vi "NR Example.vi"() -> ()   [LabVIEW 2016]
uses:
  Source/SA/RFmxNR/Typedefs/NR Common Configuration.ctl
  Source/SA/RFmxNR/Typedefs/NR Signal Configuration.ctl
  Source/SA/RFmxNR/Typedefs/NR ModAcc Configuration.ctl
  Source/SA/RFmxNR/Typedefs/NR ACP Configuration.ctl
  Source/SA/RFmxNR/Typedefs/NR ModAcc Results.ctl
  Source/SA/RFmxNR/Typedefs/NR ModAcc Component Carrier Results.ctl
  Source/SA/RFmxNR/Typedefs/NR ACP Results.ctl
  Source/SA/RFmxNR/Typedefs/NR ACP Offset Results.ctl
  Source/SA/RFmxNR/Typedefs/NR ACP Component Carrier Results.ctl
  Source/SA/RFmxNR/Typedefs/NR CHP Configuration.ctl
  Source/SA/RFmxNR/Typedefs/NR CHP Results.ctl
  Source/SA/RFmxNR/Typedefs/NR CHP Component Carrier Results.ctl
  Source/SA/RFmxNR/RFmxNR.lvlib
panel:
  out "CHP Results":T1
  out "error out":errorcluster
  out "ACP Results":T3
  out "ModAcc Results":T6
  in  "Tab Control":T8(tab)=enum."CHP"
  in  "Common Configuration":T9={"Center Frequency (Hz)"=3500000000.0, "Reference Level (dBm)"=0.0, "External Attenuation (dB)"=0.0, "Frequency Reference Source"="PXI_Clk", "Enable Trigger?"=TRUE, "Digital Edge Source"="PXI_Trig0", "Digital Edge Type"=0, "Trigger Delay (s)"=0.0, "Auto Level Enabled?"=FALSE, "Auto Level Measurement Interval (s)"=0.01} {"Auto Level Measurement Interval (s)" format="%.3p"; "Trigger Delay (s)" format="%.3p"; "Digital Edge Type" items=["Rising Edge", "Falling Edge"]; "External Attenuation (dB)" format="%.2f"; "Reference Level (dBm)" format="%.2f"; "Center Frequency (Hz)" format="%.6p"}
  in  "Resource Name":refnum<k15>="VST2_01"
  in  "Signal Configuration":T10={"Link Direction"=1, "Frequency Range"=0, "Band"=78, "Auto Resource Block Detection Enabled"=1, "Component Carrier Configurations"=[{"Bandwidth (Hz)"=100000000.0, "Cell ID"=0, "PUSCH Modulation Type"=1, "Subcarrier Spacing (Hz)"=30000.0, "PUSCH Resource Block Offset"=0, "PUSCH Number of Resource Blocks"=-1, "PUSCH Transform Precoding Enabled"=0, "PUSCH Slot Allocation"="0-Last", "PUSCH Symbol Allocation"="0-Last", "PUSCH DMRS Configuration Type"=0, "PUSCH Mapping Type"=0, "PUSCH DMRS Type A Position"=2, "PUSCH DMRS Duration"=1, "PUSCH DMRS Additional Positions"=0}]} {"Component Carrier Configurations"."PUSCH DMRS Additional Positions" items=["0", "1", "2", "3"]; "Component Carrier Configurations"."PUSCH DMRS Duration" items=["Single-Symbol"=1, "Double-Symbol"=2]; "Component Carrier Configurations"."PUSCH DMRS Type A Position" items=["2"=2, "3"=3]; "Component Carrier Configurations"."PUSCH Mapping Type" items=["Type A", "Type B"]; "Component Carrier Configurations"."PUSCH DMRS Configuration Type" items=["Type 1", "Type 2"]; "Component Carrier Configurations"."PUSCH Transform Precoding Enabled" items=["False", "True"]; "Component Carrier Configurations"."Subcarrier Spacing (Hz)" items=["15kHz"=15000.0, "30kHz"=30000.0, "60kHz"=60000.0, "120kHz"=120000.0]; "Component Carrier Configurations"."PUSCH Modulation Type" items=["PI/2 BPSK", "QPSK", "16 QAM", "64 QAM", "256 QAM"]; "Component Carrier Configurations"."Bandwidth (Hz)" items=["5M"=5000000.0, "10M"=10000000.0, "15M"=15000000.0, "20M"=20000000.0, "25M"=25000000.0, "30M"=30000000.0, "40M"=40000000.0, "50M"=50000000.0, "60M"=60000000.0, "70M"=70000000.0, "80M"=80000000.0, "90M"=90000000.0, "100M"=100000000.0, "200M"=200000000.0, "400M"=400000000.0]; "Auto Resource Block Detection Enabled" items=["False", "True"]; "Frequency Range" items=["Range 1", "Range 2"]; "Link Direction" items=["Downlink", "Uplink"]}
  in  "ACP Configuration":T11={"Number of UTRA Offsets"=2, "Number of EUTRA Offsets"=0, "Number of NR Offsets"=1, "Number of ENDC Offsets"=0, "Measurement Method"=0, "Noise Compensation Enabled"=0, "Sweep Time Auto"=1, "Sweep Time Interval (s)"=0.001, "Averaging Enabled"=0, "Averaging Count"=10, "Averaging Type"=0} {"Measurement Method" items=["Normal", "Dynamic Range", "Sequential FFT"]; "Noise Compensation Enabled" items=["False", "True"]; "Sweep Time Auto" items=["False", "True"]; "Averaging Type" items=["RMS", "Log", "Scalar", "Max", "Min"]; "Averaging Enabled" items=["False", "True"]}
  in  "ModAcc Configuration":T12={"Measurement Length Unit"=1, "Measurement Offset"=0.0, "Measurement Length"=1.0, "EVM Unit"=0, "Averaging Enabled"=0, "Averaging Count"=10} {"Averaging Enabled" items=["False", "True"]; "EVM Unit" items=["Percentage", "dB"]; "Measurement Length Unit" items=["Slot"=1, "Subframe"=3, "Time"=6]}
  in  "CHP Configuration":T13={"Sweep Time Auto"=1, "Sweep Time Interval (s)"=0.001, "Averaging Enabled"=0, "Averaging Count"=10, "Averaging Type"=0} {"Sweep Time Auto" items=["False", "True"]; "Averaging Type" items=["RMS", "Log", "Scalar", "Max", "Min"]; "Averaging Enabled" items=["False", "True"]}
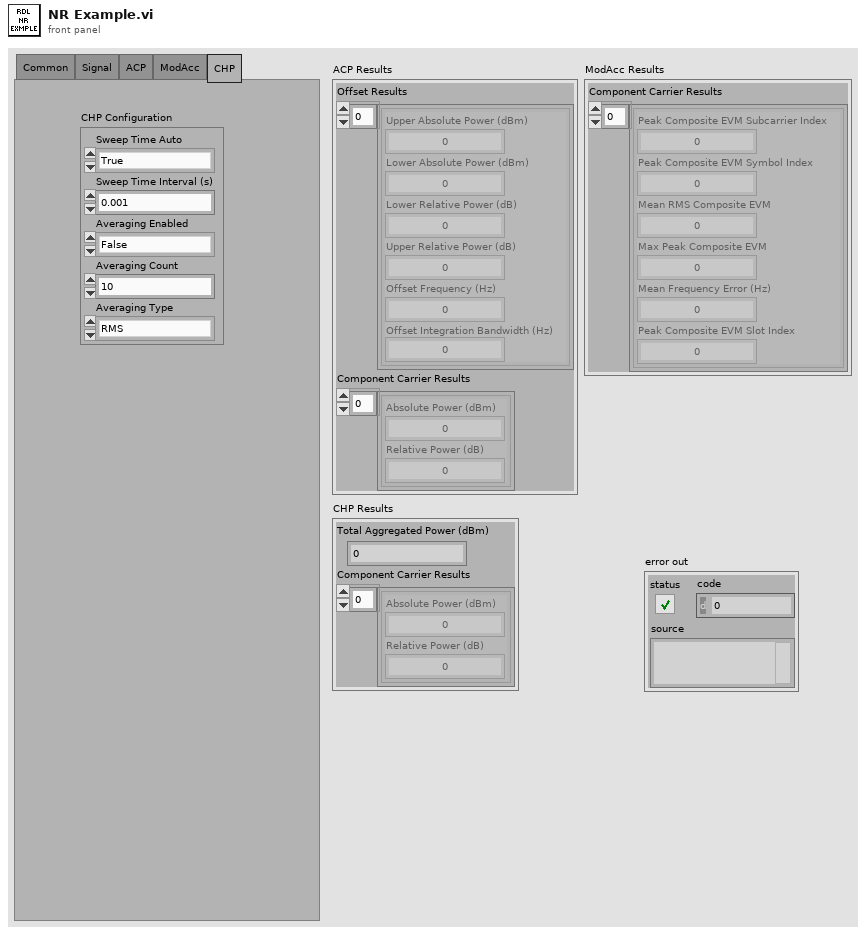
[diagram p1: front panel]
types:
  T1 = typedef "RFmxNR.lvlib/NR CHP Results.ctl" = cluster{"Total Aggregated Power (dBm)":dbl, "Component Carrier Results":T2[]}
  T2 = typedef "RFmxNR.lvlib/NR CHP Component Carrier Results.ctl" = cluster{"Absolute Power (dBm)":dbl, "Relative Power (dB)":dbl}
  T3 = typedef "RFmxNR.lvlib/NR ACP Results.ctl" = cluster{"Offset Results":T4[], "Component Carrier Results":T5[]}
  T4 = typedef "RFmxNR.lvlib/NR ACP Offset Results.ctl" = cluster{"Upper Absolute Power (dBm)":dbl, "Lower Absolute Power (dBm)":dbl, "Lower Relative Power (dB)":dbl, "Upper Relative Power (dB)":dbl, "Offset Frequency (Hz)":dbl, "Offset Integration Bandwidth (Hz)":dbl}
  T5 = typedef "RFmxNR.lvlib/NR ACP Component Carrier Results.ctl" = cluster{"Absolute Power (dBm)":dbl, "Relative Power (dB)":dbl}
  T6 = typedef "RFmxNR.lvlib/NR ModAcc Results.ctl" = cluster{"Component Carrier Results":T7[]}
  T7 = typedef "RFmxNR.lvlib/NR ModAcc Component Carrier Results.ctl" = cluster{"Peak Composite EVM Subcarrier Index":i32, "Peak Composite EVM Symbol Index":i32, "Mean RMS Composite EVM":dbl, "Max Peak Composite EVM":dbl, "Mean Frequency Error (Hz)":dbl, "Peak Composite EVM Slot Index":i32}
  T8 = enum32{"Common", "Signal", "ACP", "ModAcc", "CHP"}
  T9 = typedef "RFmxNR.lvlib/NR Common Configuration.ctl" = cluster{"Center Frequency (Hz)":dbl, "Reference Level (dBm)":dbl, "External Attenuation (dB)":dbl, "Frequency Reference Source":string, "Enable Trigger?":bool, "Digital Edge Source":string, "Digital Edge Type":i32, "Trigger Delay (s)":dbl, "Auto Level Enabled?":bool, "Auto Level Measurement Interval (s)":dbl}
  T10 = typedef "RFmxNR.lvlib/NR Signal Configuration.ctl" = cluster{"Link Direction":i32, "Frequency Range":i32, "Band":i32, "Auto Resource Block Detection Enabled":i32, "Component Carrier Configurations":cluster{"Bandwidth (Hz)":dbl, "Cell ID":i32, "PUSCH Modulation Type":i32, "Subcarrier Spacing (Hz)":dbl, "PUSCH Resource Block Offset":i32, "PUSCH Number of Resource Blocks":i32, "PUSCH Transform Precoding Enabled":i32, "PUSCH Slot Allocation":string, "PUSCH Symbol Allocation":string, "PUSCH DMRS Configuration Type":i32, "PUSCH Mapping Type":i32, "PUSCH DMRS Type A Position":i32, "PUSCH DMRS Duration":i32, "PUSCH DMRS Additional Positions":i32}[]}
  T11 = typedef "RFmxNR.lvlib/NR ACP Configuration.ctl" = cluster{"Number of UTRA Offsets":i32, "Number of EUTRA Offsets":i32, "Number of NR Offsets":i32, "Number of ENDC Offsets":i32, "Measurement Method":i32, "Noise Compensation Enabled":i32, "Sweep Time Auto":i32, "Sweep Time Interval (s)":dbl, "Averaging Enabled":i32, "Averaging Count":i32, "Averaging Type":i32}
  T12 = typedef "RFmxNR.lvlib/NR ModAcc Configuration.ctl" = cluster{"Measurement Length Unit":i32, "Measurement Offset":dbl, "Measurement Length":dbl, "EVM Unit":i32, "Averaging Enabled":i32, "Averaging Count":i32}
  T13 = typedef "RFmxNR.lvlib/NR CHP Configuration.ctl" = cluster{"Sweep Time Auto":i32, "Sweep Time Interval (s)":dbl, "Averaging Enabled":i32, "Averaging Count":i32, "Averaging Type":i32}
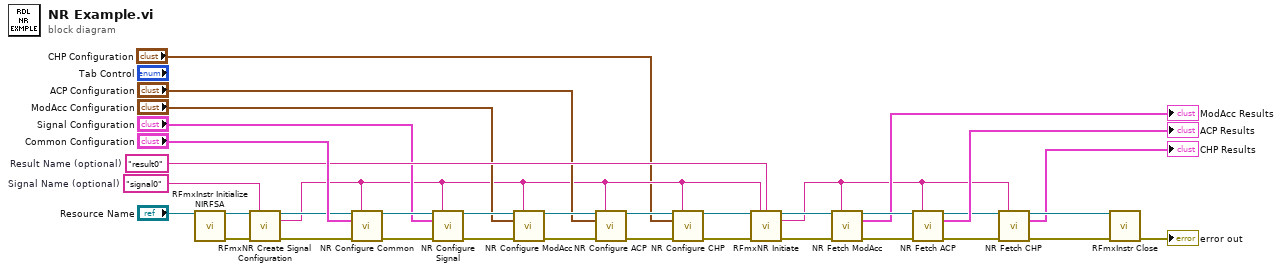
[diagram p0: block diagram]
diagram:
  w15 = "result0"  # Result Name (optional)
  w16 = "signal0"  # Signal Name (optional)
  n1 = call <vilib>:"RFmxInstr Initialize NIRFSA.vi"("Resource Name"="Resource Name") -> ("Instrument Handle Out"=w18:refnum<k21>, "error out"=w34:errorcluster)  [unwired: 12 in, 1 out]
  n2 = call <vilib>:"RFmxNR Create Signal Configuration.vi"("Instrument Handle In"=w18, "Signal Name"=w16, "error in (no error)"=w34) -> ("Instrument Handle Out"=w17:refnum<k21>, "Selector String Out"=w7:string, "error out"=w19:errorcluster)  [unwired: 10 in]
  n3 = call "NR Configure Common.vi"("RFmx Handle In"=w17, "Selector String"=w7, "NR Common Configuration"="Common Configuration", "error in (no error)"=w19) -> ("RFmx Handle Out"=w36:refnum<k21>, "error out"=w35:errorcluster)  [unwired: 10 in]
  n4 = call "NR Configure Signal.vi"("RFmx Handle In"=w36, "Selector String"=w7, "NR Signal Configuration"="Signal Configuration", "error in (no error)"=w35) -> ("RFmx Handle Out"=w31:refnum<k21>, "error out"=w30:errorcluster)  [unwired: 10 in]
  n5 = call "NR Configure ModAcc.vi"("RFmx Handle In"=w31, "Selector String"=w7, "NR ModAcc Configuration"="ModAcc Configuration", "error in (no error)"=w30) -> ("RFmx Handle Out"=w29:refnum<k21>, "error out"=w28:errorcluster)  [unwired: 10 in]
  n6 = call "NR Configure ACP.vi"("RFmx Handle In"=w29, "Selector String"=w7, "NR ACP Configuration"="ACP Configuration", "error in (no error)"=w28) -> ("RFmx Handle Out"=w9:refnum<k21>, "error out"=w27:errorcluster)  [unwired: 10 in]
  n7 = call "NR Configure CHP.vi"("RFmx Handle In"=w9, "Selector String"=w7, "NR CHP Configuration"="CHP Configuration", "error in (no error)"=w27) -> ("RFmx Handle Out"=w8:refnum<k21>, "error out"=w10:errorcluster)  [unwired: 10 in]
  n8 = call <vilib>:"RFmxNR Initiate.vi"("Instrument Handle In"=w8, "Selector String"=w7, "Result Name"=w15, "error in (no error)"=w10) -> ("Instrument Handle Out"=w26:refnum<k21>, "Selector String Out"=w2:string, "error out"=w25:errorcluster)  [unwired: 9 in]
  n9 = call "NR Fetch ModAcc.vi"("RFmx Handle In"=w26, "Selector String"=w2, "error in (no error)"=w25) -> ("RFmx Handle Out"=w24:refnum<k21>, "ModAcc Results"=→"ModAcc Results":T6, "error out"=w14:errorcluster)  [unwired: 10 in]
  n10 = call "NR Fetch ACP.vi"("RFmx Handle In"=w24, "Selector String"=w2, "error in (no error)"=w14) -> ("RFmx Handle Out"=w4:refnum<k21>, "ACP Results"=→"ACP Results":T3, "error out"=w21:errorcluster)  [unwired: 10 in]
  n11 = call "NR Fetch CHP.vi"("RFmx Handle In"=w4, "Selector String"=w2, "error in (no error)"=w21) -> ("RFmx Handle Out"=w3:refnum<k21>, "CHP Results"=→"CHP Results":T1, "error out"=w5:errorcluster)  [unwired: 10 in]
  n12 = call <vilib>:"RFmxInstr Close.vi"("Instrument Handle In"=w3, "error in (no error)"=w5) -> ("error out"=→"error out":errorcluster)  [unwired: 13 in]
